vi "Columns Dictionary.vi"(0 "Action":T1, 5 "Column Header":string, 9 "Column Index":i32=-1) -> (4 "Column Index":i32, 6 "Column already included? / Column not found?":bool, 10 "Columns":cluster{string, i32}[](array[cluster]))   [LabVIEW 2023, in "RFCalAndFixtureCharact.Common.lvlib"]
uses:
  RFCalAndFixtureCharact.Common.lvlib
  Type Definitions/Dictionary Operation.ctl
  <vilib>/Utility/miscctls.llb/LVMapReplaceAction.ctl
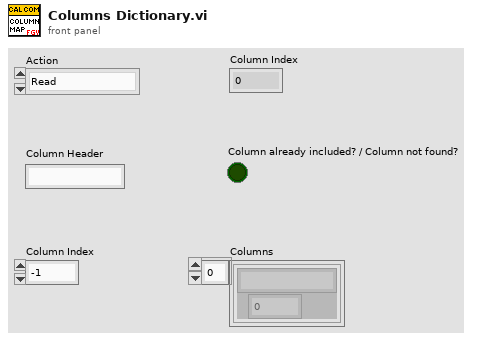
[diagram p1: front panel]
types:
  T1 = typedef "RFCalAndFixtureCharact.Common.lvlib/Dictionary Operation.ctl" = enum16{"Read", "Insert", "Remove", "Clear", "Get All", "Update"}
  T2 = typedef "LVMapReplaceAction.ctl" = enum32{"Modify Entry only if found", "Add or Modify Entry", "Delete Entry"}
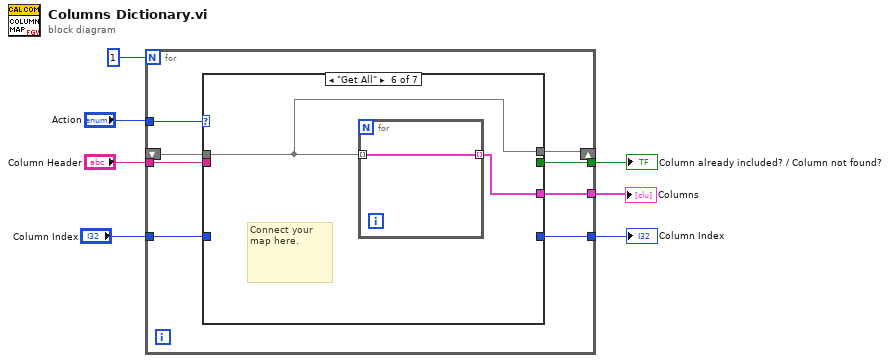
[diagram p0: block diagram]
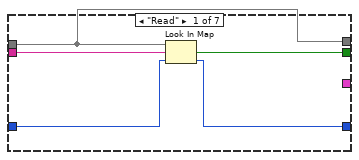
[diagram p2: hidden frame]
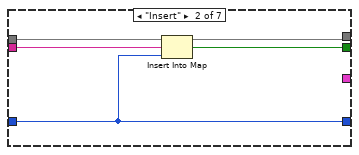
[diagram p3: hidden frame]
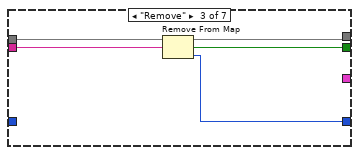
[diagram p4: hidden frame]
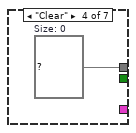
[diagram p5: hidden frame]
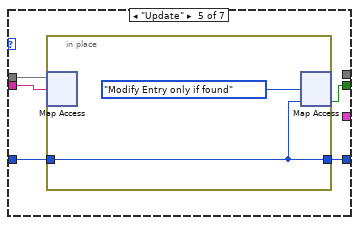
[diagram p6: hidden frame]
diagram:
  n1 = for {
    N: 1 -> [_]
    tunnel: "Action" -> [w15]
    tunnel: "Column Header" -> [w14]
    tunnel: [w13] -> w5
    tunnel: [w12] -> w2
    shift-right: [w9] -> _
    shift-left: _ -> [w11]
    tunnel: "Column Index" -> [w10]
    tunnel: [w8] -> w1
    n2 = case shown="\"Get All\"" w15 {
      tunnel: w14 -> [w20 w25 w29 _ w35 _ _]
      tunnel: w11 -> [w16 w22 w27 _ w36 w40 w43]
      tunnel: [w19 w24 w30 _ w33 _ _] -> w13
      tunnel: [w17 w23 w28 _ w32 _ w42] -> w12
      tunnel: w10 -> [w18 w23 _ _ w34 _ w42]
      tunnel: [w16 w21 w26 w31 _ w40 w43] -> w9
      tunnel: [_ _ _ _ _ w39 _] -> w8
      frame "Read" {
        n3 = Look In Map(map=w16, key=w20, default value=w18) -> (key not found?=w19:bool, value=w17:i32)
      }
      frame "Insert" {
        n4 = Insert Into Map(map in=w22, key=w25, value=w23) -> (map out=w21:map{string, i32}, key already included?=w24:bool)  [unwired: 1 out]
      }
      frame "Remove" {
        n5 = Remove From Map(10:w29, 11:w27) -> (1:w28:i32, 2:w30:bool, 3:w26:map{string, i32})
      }
      frame "Clear" {
        w31 = map{string, i32} {}  # Size: 0
      }
      frame "Update" {
        n6 = in-place {
          in-place-border: w34 -> [w37]
          in-place-border: [w37] -> w32
          n7 = in-place-map #1(w36, w35) -> ()  [unwired: 1 in, 2 out]
          n8 = in-place-map #1(w37, LVMapReplaceAction."Modify Entry only if found" ("action")) -> (w33:bool)  [unwired: 2 out]
        }
      }
      frame "Get All" {
        # "Connect your map here."
        n9 = for {
          tunnel: [w41] -> w39 mode=indexing
          tunnel: w40 -> [w41] mode=indexing
        }
      }
      frame Default {
      }
    }
  }
  "Column already included? / Column not found?" <- w5
  "Column Index" <- w2
  "Columns" <- w1
